vi "Filter_Evaluator.vi"(7 "Headers":string[](array[string])=["Packet Number", "Timestamp", "Source", "Destination", "Protocol", "Length", "Data"], 8 "Error":errorcluster, 9 "Comparators":T1(array[cluster]), 10 "Boolean Connectors":string[](array[string])=["AND", "OR"], 11 "Prefiltered Data":string[][](array[string])=array1500x7[10500 elements]) -> (0 "Error Out":errorcluster, 2 "Filtered Array":string[][](array[string]), 3 "Prefiltered Data":string[][](array[string]))   [LabVIEW 2025, in "Table_Filtering.lvlib"]
uses:
  Table_Filtering.lvlib
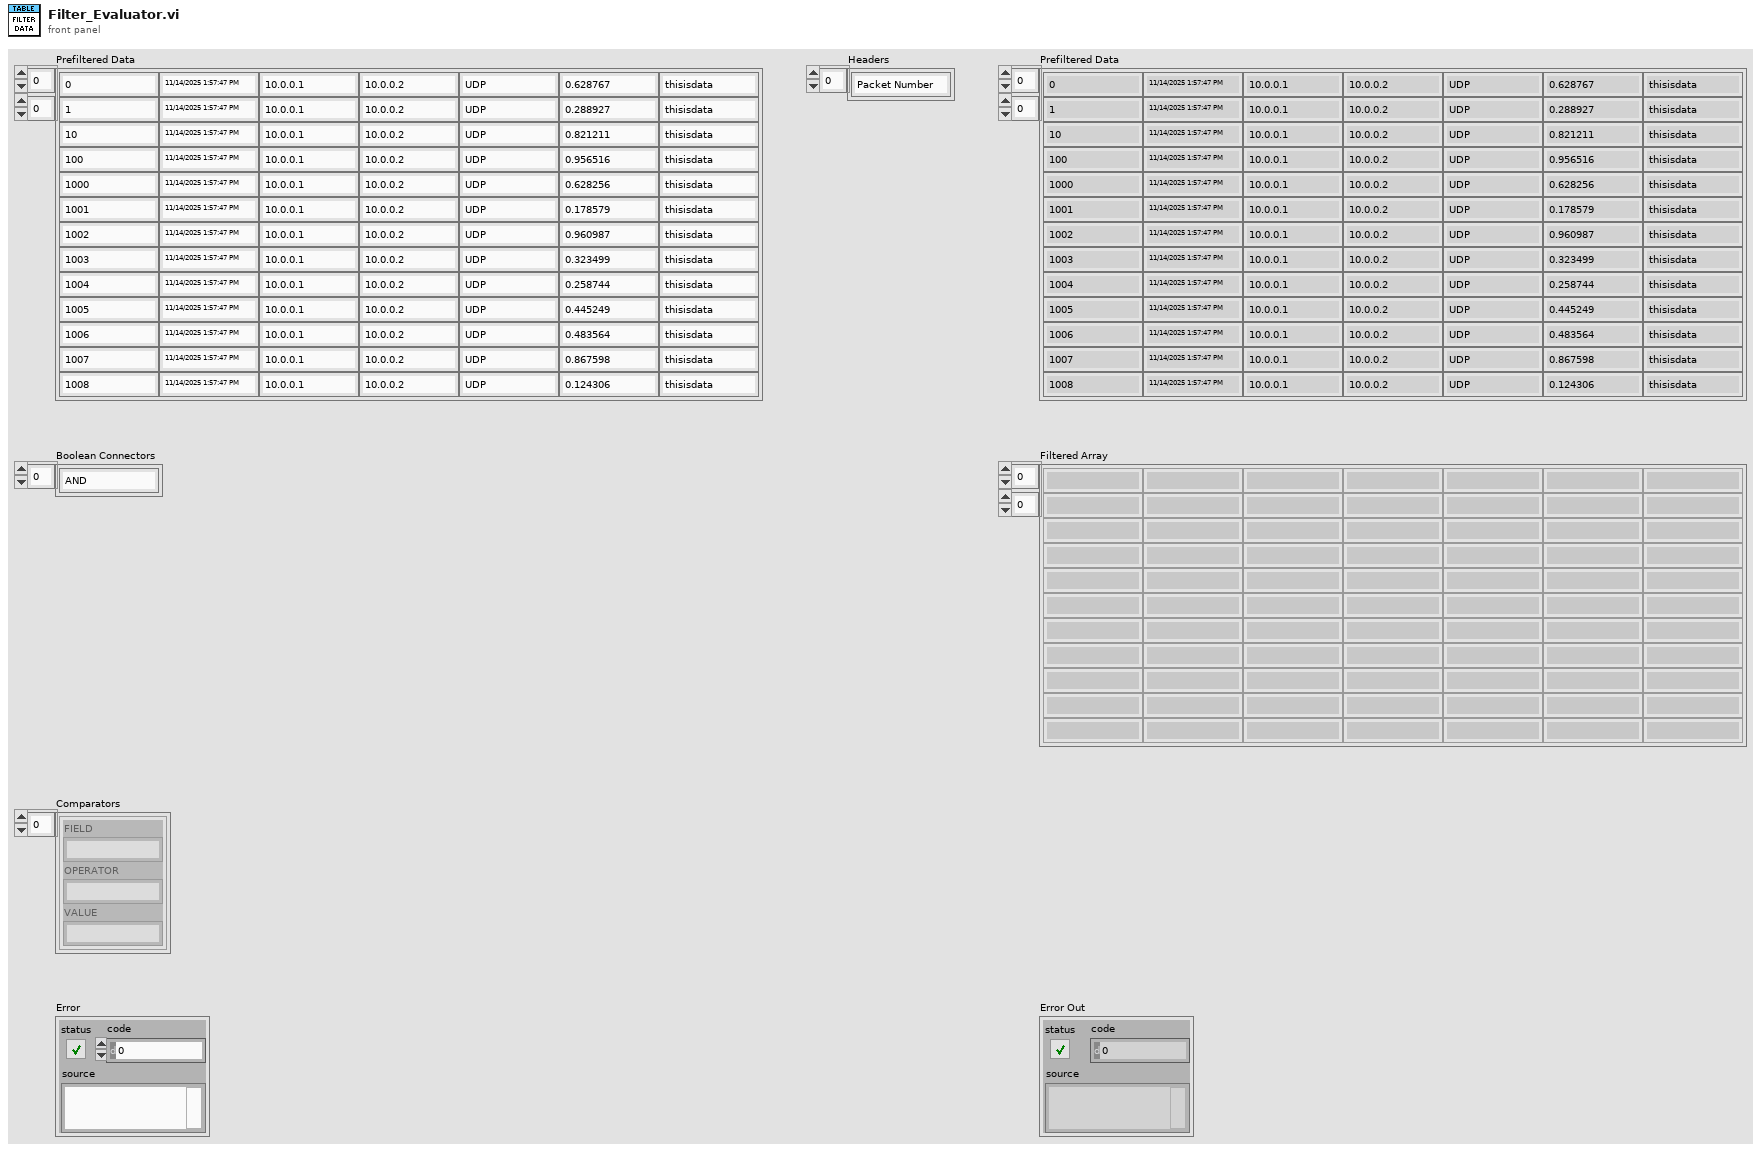
[diagram p1: front panel]
types:
  T1 = cluster{"FIELD":string, "OPERATOR":string, "VALUE":string}[]
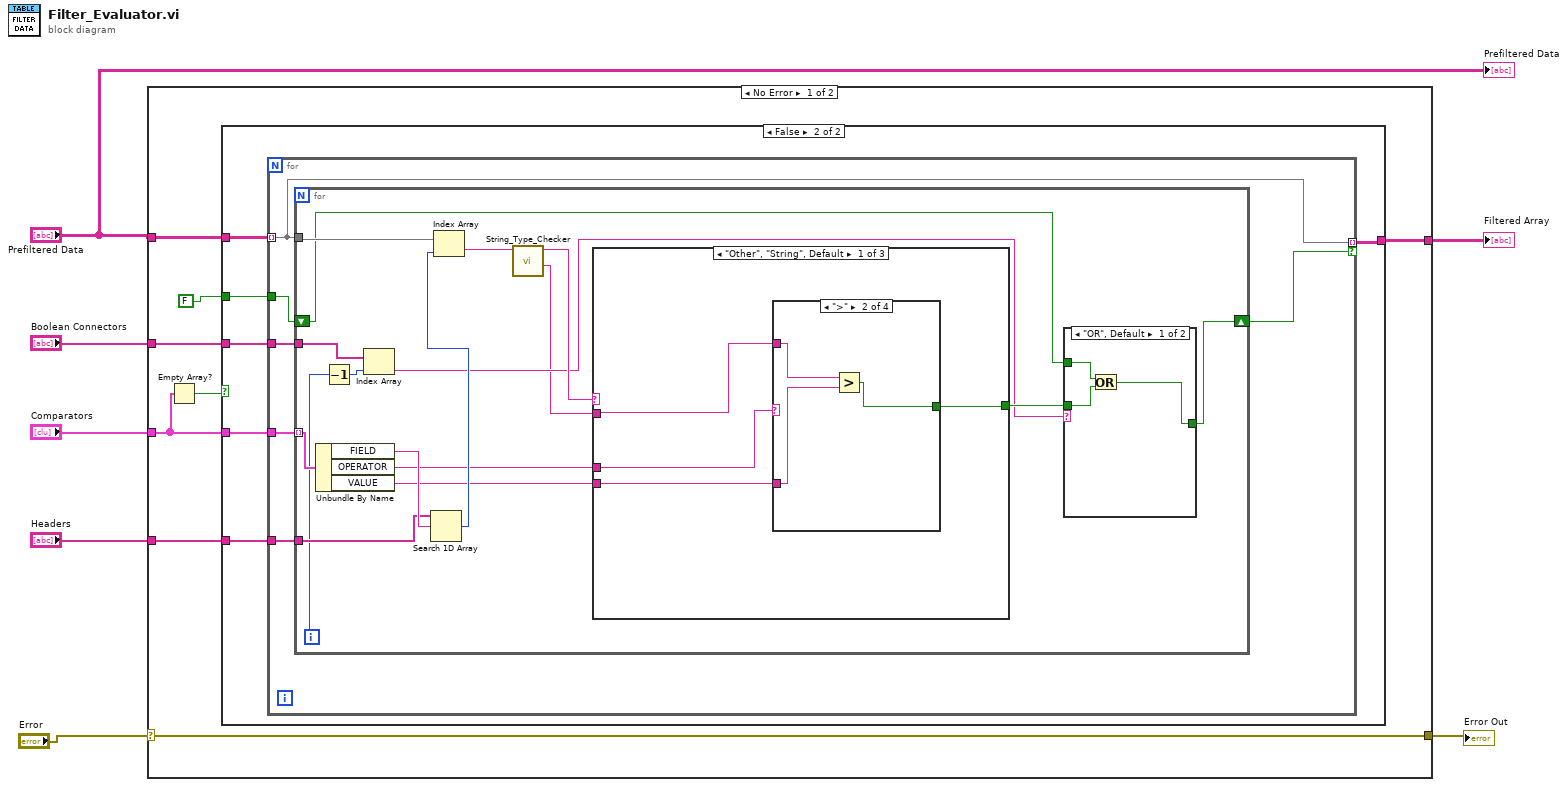
[diagram p0: block diagram]
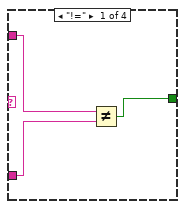
[diagram p3: hidden frame]
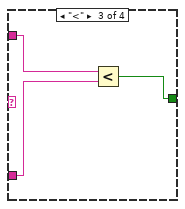
[diagram p4: hidden frame]
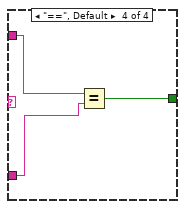
[diagram p5: hidden frame]
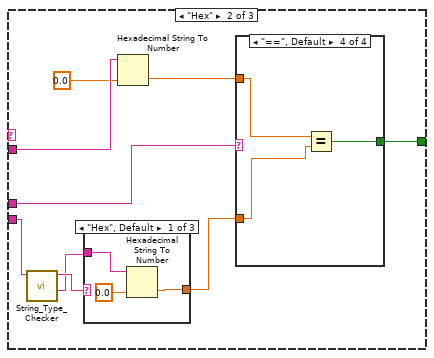
[diagram p6: hidden frame]
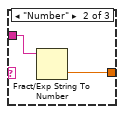
[diagram p7: hidden frame]
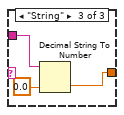
[diagram p8: hidden frame]
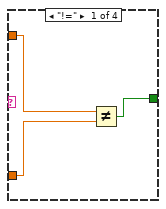
[diagram p9: hidden frame]
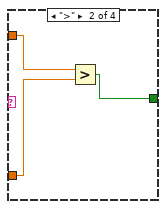
[diagram p10: hidden frame]
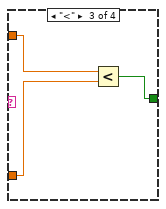
[diagram p11: hidden frame]
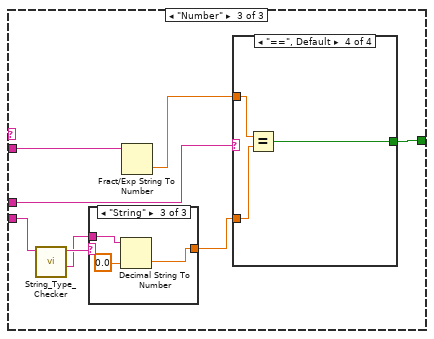
[diagram p12: hidden frame]
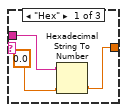
[diagram p13: hidden frame]
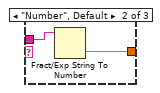
[diagram p14: hidden frame]
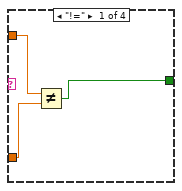
[diagram p15: hidden frame]
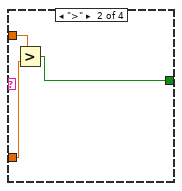
[diagram p16: hidden frame]
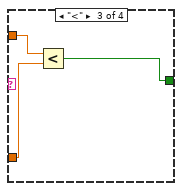
[diagram p17: hidden frame]
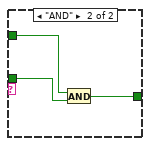
[diagram p18: hidden frame]
diagram:
  n1 = case shown="No Error" "Error" {
    selector: "Error" -> [w11 w125]
    tunnel: "Headers" -> [w15 _]
    tunnel: "Boolean Connectors" -> [w14 _]
    tunnel: "Comparators" -> [w8 _]
    tunnel: "Prefiltered Data" -> [w13 _]
    tunnel: [w12 _] -> w7
    tunnel: [w11 w125] -> w2
    frame No Error {
      n2 = Empty Array?(array=w8) -> (empty?=w9:bool)
      n3 = case shown="False" w9 {
        tunnel: w15 -> [_ w22]
        tunnel: FALSE -> [_ w21]
        tunnel: w14 -> [_ w20]
        tunnel: w8 -> [_ w19]
        tunnel: w13 -> [w16 w18]
        tunnel: [w16 w17] -> w12
        frame True {
        }
        frame False {
          n4 = for {
            tunnel: w22 -> [w28]
            tunnel: w19 -> [w27]
            tunnel: w18 -> [w23] mode=indexing
            tunnel: w21 -> [w26]
            tunnel: w20 -> [w25]
            tunnel: [w23] -> w17 mode=indexing if=w24
            n5 = for {
              tunnel: w28 -> [w42]
              tunnel: w27 -> [w45] mode=indexing
              tunnel: w23 -> [w44]
              shift-right: [w36] -> w24
              shift-left: w26 -> [w37]
              tunnel: w25 -> [w40]
              i -> [w38]
              n6 = Unbundle By Name(w45) -> ("FIELD"=w43:string, "OPERATOR"=w32:string, "VALUE"=w33:string)
              n7 = Decrement(x=w38) -> (x-1=w39:i32)
              n8 = Index Array(array=w40, index=w39) -> (element=w30:string)
              n9 = Search 1D Array(1D array=w42, element=w43) -> (index of element=w41:i32)  [unwired: 1 in]
              n10 = Index Array(array=w44, index=w41) -> (element=w34:string)
              n11 = call "String_Type_Checker.vi"("String"=w34) -> ("Number"=w29:string, "Type"=w35:string)  [unwired: 9 in]
              n12 = case shown="\"Other\", \"String\", Default" w35 {
                tunnel: w29 -> [w49 w70 w98]
                tunnel: w33 -> [w46 w65 w94]
                tunnel: w32 -> [w48 w68 w97]
                tunnel: [w47 w67 w96] -> w31
                frame "Other", "String", Default {
                  n13 = case shown="\">\"" w48 {
                    tunnel: w49 -> [w51 w55 w58 w59]
                    tunnel: w46 -> [w50 w54 w57 w61]
                    tunnel: [w52 w53 w56 w60] -> w47
                    frame "!=" {
                      n14 = Not Equal?(x=w51, y=w50) -> (x != y?=w52:bool)
                    }
                    frame ">" {
                      n15 = Greater?(x=w55, y=w54) -> (0:w53:bool)
                    }
                    frame "<" {
                      n16 = Less?(x=w58, y=w57) -> (x < y?=w56:bool)
                    }
                    frame "==", Default {
                      n17 = Equal?(x=w59, y=w61) -> (x = y?=w60:bool)
                    }
                  }
                }
                frame "Hex" {
                  n18 = call "String_Type_Checker.vi"("String"=w65) -> ("Number"=w62:string, "Type"=w63:string)  [unwired: 9 in]
                  n19 = case shown="\"Hex\", Default" w63 {
                    tunnel: [w71 w75 w78] -> w66
                    tunnel: w62 -> [w73 w74 w76]
                    frame "Hex", Default {
                      n20 = Hexadecimal String To Number(string=w73, default (0uL)=0.0) -> (number=w71:dbl)  [unwired: 1 in, 1 out]
                    }
                    frame "Number" {
                      n21 = Fract/Exp String To Number(string=w74) -> (number=w75:dbl)  [unwired: 3 in, 1 out]
                    }
                    frame "String" {
                      n22 = Decimal String To Number(string=w76, default (0L)=0.0) -> (number=w78:dbl)  [unwired: 1 in, 1 out]
                    }
                  }
                  n23 = Hexadecimal String To Number(string=w70, default (0uL)=0.0) -> (number=w69:dbl)  [unwired: 1 in, 1 out]
                  n24 = case shown="\"==\", Default" w68 {
                    tunnel: w69 -> [w80 w84 w87 w88]
                    tunnel: w66 -> [w79 w83 w86 w90]
                    tunnel: [w81 w82 w85 w89] -> w67
                    frame "!=" {
                      n25 = Not Equal?(x=w80, y=w79) -> (x != y?=w81:bool)
                    }
                    frame ">" {
                      n26 = Greater?(x=w84, y=w83) -> (0:w82:bool)
                    }
                    frame "<" {
                      n27 = Less?(x=w87, y=w86) -> (x < y?=w85:bool)
                    }
                    frame "==", Default {
                      n28 = Equal?(x=w88, y=w90) -> (x = y?=w89:bool)
                    }
                  }
                }
                frame "Number" {
                  n29 = call "String_Type_Checker.vi"("String"=w94) -> ("Number"=w92:string, "Type"=w93:string)  [unwired: 9 in]
                  n30 = case shown="\"String\"" w93 {
                    tunnel: [w99 w103 w106] -> w91
                    tunnel: w92 -> [w101 w102 w104]
                    frame "Hex" {
                      n31 = Hexadecimal String To Number(string=w101, default (0uL)=0.0) -> (number=w99:dbl)  [unwired: 1 in, 1 out]
                    }
                    frame "Number", Default {
                      n32 = Fract/Exp String To Number(string=w102) -> (number=w103:dbl)  [unwired: 3 in, 1 out]
                    }
                    frame "String" {
                      n33 = Decimal String To Number(string=w104, default (0L)=0.0) -> (number=w106:dbl)  [unwired: 1 in, 1 out]
                    }
                  }
                  n34 = Fract/Exp String To Number(string=w98) -> (number=w95:dbl)  [unwired: 3 in, 1 out]
                  n35 = case shown="\"==\", Default" w97 {
                    tunnel: w91 -> [w108 w112 w115 w118]
                    tunnel: [w109 w111 w114 w117] -> w96
                    tunnel: w95 -> [w107 w110 w113 w116]
                    frame "!=" {
                      n36 = Not Equal?(x=w107, y=w108) -> (x != y?=w109:bool)
                    }
                    frame ">" {
                      n37 = Greater?(x=w110, y=w112) -> (0:w111:bool)
                    }
                    frame "<" {
                      n38 = Less?(x=w113, y=w115) -> (x < y?=w114:bool)
                    }
                    frame "==", Default {
                      n39 = Equal?(x=w116, y=w118) -> (x = y?=w117:bool)
                    }
                  }
                }
              }
              n40 = case shown="\"OR\", Default" w30 {
                tunnel: w37 -> [w120 w124]
                tunnel: [w121 w123] -> w36
                tunnel: w31 -> [w119 w122]
                frame "OR", Default {
                  n41 = Or(x=w120, y=w119) -> (x .or. y?=w121:bool)
                }
                frame "AND" {
                  n42 = And(x=w124, y=w122) -> (x .and. y?=w123:bool)
                }
              }
            }
          }
        }
      }
    }
    frame Error {
    }
  }
  "Filtered Array" <- w7
  "Error Out" <- w2
  "Prefiltered Data" <- "Prefiltered Data"
